vi "Nested Malleable VIs - Lesson 5.vi"() -> ()   [LabVIEW 2023]
doc: "Lesson 5 explores how creating nested VIMs can improve your code reuse, allowing many different malleable algorithms to be built around the same malleable core."
uses:
  Numeric Strings Less Functor/Numeric Strings Less Functor.lvclass
  e3db7b28-214a-4d56-9631-a08b30ab005c.vi
  c33f52e0-d72d-45e0-ba34-8b6af2d75d3b.vi
  2e45c285-a169-4a6c-a5e0-64cd902b0f72.vi
  f9130e0b-cd9d-4b76-83ef-857f5d1a4067.vi
  e3db7b28-214a-4d56-9631-a08b30ab005c.vi/4611cae3-c7be-41e2-9a5e-ea0ae78a7ced.vi
  c33f52e0-d72d-45e0-ba34-8b6af2d75d3b.vi/c0db33a9-eb6c-44d9-b982-8563e05d2734.vi
  c33f52e0-d72d-45e0-ba34-8b6af2d75d3b.vi/ae3535a8-0066-4e8d-a5de-b07ac05a7c65.vi
  c33f52e0-d72d-45e0-ba34-8b6af2d75d3b.vi/dda8e586-731b-4197-ad83-6a4d05585a0a.vi
  2e45c285-a169-4a6c-a5e0-64cd902b0f72.vi/4611cae3-c7be-41e2-9a5e-ea0ae78a7ced.vi
  f9130e0b-cd9d-4b76-83ef-857f5d1a4067.vi/d4db2432-cc9c-482c-8957-dac855435ef6.vi
  f9130e0b-cd9d-4b76-83ef-857f5d1a4067.vi/86fbf154-bd7b-49a2-8ab2-a837b2a95f24.vi
  f9130e0b-cd9d-4b76-83ef-857f5d1a4067.vi/3b95b01e-1ec2-4565-bcd9-7606a5281010.vi
  f9130e0b-cd9d-4b76-83ef-857f5d1a4067.vi/96a08935-737a-44b2-979c-a81d56408f7e.vi
  e3db7b28-214a-4d56-9631-a08b30ab005c.vi/4611cae3-c7be-41e2-9a5e-ea0ae78a7ced.vi/19e2e4cb-e3bb-4239-bd5f-680916605f5d.vi
  e3db7b28-214a-4d56-9631-a08b30ab005c.vi/4611cae3-c7be-41e2-9a5e-ea0ae78a7ced.vi/f72612c1-738a-48a1-9fcf-3db66cb27fb3.vi
  e3db7b28-214a-4d56-9631-a08b30ab005c.vi/4611cae3-c7be-41e2-9a5e-ea0ae78a7ced.vi/45406051-8994-464b-8b47-ac12a8cbadfa.vi
  e3db7b28-214a-4d56-9631-a08b30ab005c.vi/4611cae3-c7be-41e2-9a5e-ea0ae78a7ced.vi/dd886480-778c-48b1-8e4a-d6890e1a60dd.vi
  e3db7b28-214a-4d56-9631-a08b30ab005c.vi/4611cae3-c7be-41e2-9a5e-ea0ae78a7ced.vi/2e6e140f-e361-4312-a09e-e37273ac7fd1.vi
  e3db7b28-214a-4d56-9631-a08b30ab005c.vi/4611cae3-c7be-41e2-9a5e-ea0ae78a7ced.vi/3589548e-4c68-4568-af05-72ab28470577.vi
  e3db7b28-214a-4d56-9631-a08b30ab005c.vi/4611cae3-c7be-41e2-9a5e-ea0ae78a7ced.vi/cf64d4f5-91bd-4749-9577-68c6ded0155b.vi
  e3db7b28-214a-4d56-9631-a08b30ab005c.vi/4611cae3-c7be-41e2-9a5e-ea0ae78a7ced.vi/6f6fefe9-f25b-4595-b26f-75715299a794.vi
  e3db7b28-214a-4d56-9631-a08b30ab005c.vi/4611cae3-c7be-41e2-9a5e-ea0ae78a7ced.vi/c74ffb76-1048-4639-9a95-b6de96ba7014.vi
  2e45c285-a169-4a6c-a5e0-64cd902b0f72.vi/4611cae3-c7be-41e2-9a5e-ea0ae78a7ced.vi/19e2e4cb-e3bb-4239-bd5f-680916605f5d.vi
  2e45c285-a169-4a6c-a5e0-64cd902b0f72.vi/4611cae3-c7be-41e2-9a5e-ea0ae78a7ced.vi/f72612c1-738a-48a1-9fcf-3db66cb27fb3.vi
  2e45c285-a169-4a6c-a5e0-64cd902b0f72.vi/4611cae3-c7be-41e2-9a5e-ea0ae78a7ced.vi/45406051-8994-464b-8b47-ac12a8cbadfa.vi
  2e45c285-a169-4a6c-a5e0-64cd902b0f72.vi/4611cae3-c7be-41e2-9a5e-ea0ae78a7ced.vi/dd886480-778c-48b1-8e4a-d6890e1a60dd.vi
  2e45c285-a169-4a6c-a5e0-64cd902b0f72.vi/4611cae3-c7be-41e2-9a5e-ea0ae78a7ced.vi/2e6e140f-e361-4312-a09e-e37273ac7fd1.vi
  2e45c285-a169-4a6c-a5e0-64cd902b0f72.vi/4611cae3-c7be-41e2-9a5e-ea0ae78a7ced.vi/3589548e-4c68-4568-af05-72ab28470577.vi
  2e45c285-a169-4a6c-a5e0-64cd902b0f72.vi/4611cae3-c7be-41e2-9a5e-ea0ae78a7ced.vi/cf64d4f5-91bd-4749-9577-68c6ded0155b.vi
  2e45c285-a169-4a6c-a5e0-64cd902b0f72.vi/4611cae3-c7be-41e2-9a5e-ea0ae78a7ced.vi/6f6fefe9-f25b-4595-b26f-75715299a794.vi
  2e45c285-a169-4a6c-a5e0-64cd902b0f72.vi/4611cae3-c7be-41e2-9a5e-ea0ae78a7ced.vi/c74ffb76-1048-4639-9a95-b6de96ba7014.vi
  f9130e0b-cd9d-4b76-83ef-857f5d1a4067.vi/d4db2432-cc9c-482c-8957-dac855435ef6.vi/6eaecd13-6e48-4772-a921-b51ebdf84d88.vi
  f9130e0b-cd9d-4b76-83ef-857f5d1a4067.vi/d4db2432-cc9c-482c-8957-dac855435ef6.vi/d2d5f2b7-06f4-47f6-971c-049c3fdbb653.vi
  f9130e0b-cd9d-4b76-83ef-857f5d1a4067.vi/3b95b01e-1ec2-4565-bcd9-7606a5281010.vi/6eaecd13-6e48-4772-a921-b51ebdf84d88.vi
  f9130e0b-cd9d-4b76-83ef-857f5d1a4067.vi/3b95b01e-1ec2-4565-bcd9-7606a5281010.vi/d2d5f2b7-06f4-47f6-971c-049c3fdbb653.vi
  f9130e0b-cd9d-4b76-83ef-857f5d1a4067.vi/96a08935-737a-44b2-979c-a81d56408f7e.vi/6eaecd13-6e48-4772-a921-b51ebdf84d88.vi
  f9130e0b-cd9d-4b76-83ef-857f5d1a4067.vi/96a08935-737a-44b2-979c-a81d56408f7e.vi/d2d5f2b7-06f4-47f6-971c-049c3fdbb653.vi
  Numeric Strings Less Functor/Less Than.vi
panel:
  out "sorted array 3":string[](array[string])
  out "sorted array 2":string[](array[string])
  out "sorted array 1":string[](array[string])
  out "found":bool
  out "nearest index":i32
  # "Overview: This lesson explores how creating nested VIMs can improve your code reuse, allowing many different algorithms to be built around the same malleable core. \n\nInstructions: \n1. Open the block diagram of this VI. Review the lessons presented there.\n2. Run the VI to see the results. \n3. This lesson concludes this example."
  # "This array is sorted by string value, ignoring case."
  # "This array is sorted by string value, ignoring case."
  # "This array is sorted by the value of the number at the front, ignoring the rest of the string."
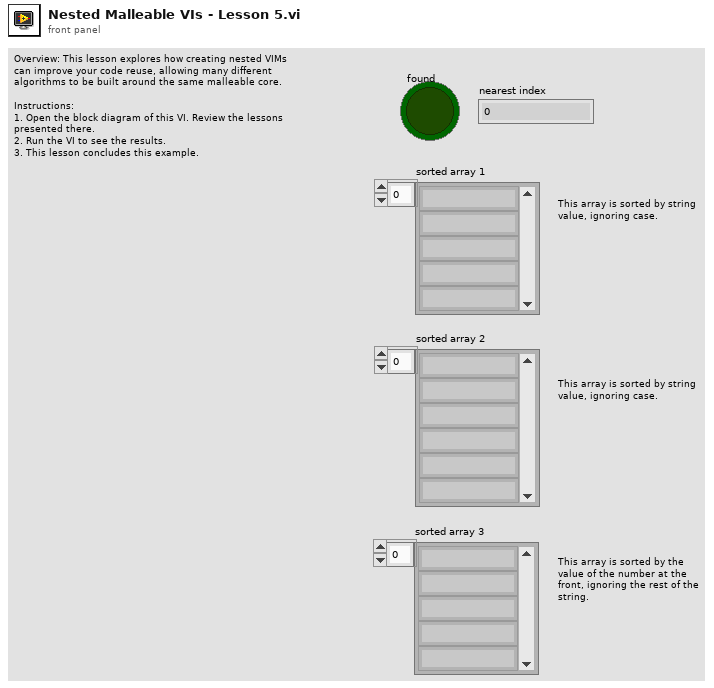
[diagram p1: front panel]
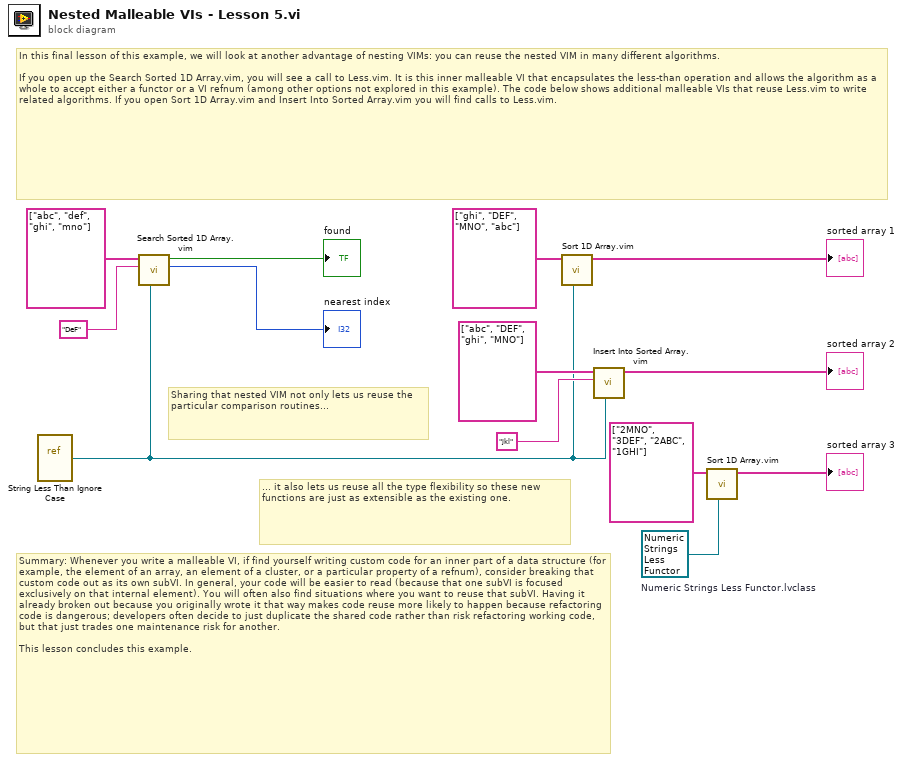
[diagram p0: block diagram]
diagram:
  w5 = refnum<class "Numeric Strings Less Functor.lvclass"> refnum  # Numeric Strings Less Functor.lvclass
  # "... it also lets us reuse all the type flexibility so these new functions are just as extensible as the existing one."
  # "Sharing that nested VIM not only lets us reuse the particular comparison routines..."
  # "Summary: Whenever you write a malleable VI, if find yourself writing custom code for an inner part of a data structure (for example, the element of an array, an element of a cluster, or a particular property of a refnum), consider breaking that custom code out as its own subVI. In general, your code will be easier to read (because that one subVI is focused exclusively on that internal element). You will often also find situations where you want to reuse that subVI. Having it already broken out because you originally wrote it that way makes code reuse more likely to happen because refactoring code is dangerous; developers often decide to just duplicate the shared code rather than risk refactoring working code, but that just trades one maintenance risk for another.\n\nThis lesson concludes this example."
  # "In this final lesson of this example, we will look at another advantage of nesting VIMs: you can reuse the nested VIM in many different algorithms.\n\nIf you open up the Search Sorted 1D Array.vim, you will see a call to Less.vim. It is this inner malleable VI that encapsulates the less-than operation and allows the algorithm as a whole to accept either a functor or a VI refnum (among other options not explored in this example). The code below shows additional malleable VIs that reuse Less.vim to write related algorithms. If you open Sort 1D Array.vim and Insert Into Sorted Array.vim you will find calls to Less.vim."
  n1 = vi-ref "String Less Than Ignore Case.vi"() -> (w1:refnum<vi>)
  n2 = call "Search Sorted 1D Array.vim"("less function (built-in <)"=w1, "element"="DeF", "sorted 1D array"=string[] ["abc", "def", "ghi", "mno"] ("1D array")) -> ("nearest index"=→"nearest index":i32, "found?"=→"found":bool)  [unwired: 7 in]
  n3 = call "Sort 1D Array.vim"("less function (built-in <)"=w1, "unsorted array"=string[] ["ghi", "DEF", "MNO", "abc"] ("1D array")) -> ("sorted array"=→"sorted array 1":string[])  [unwired: 9 in]
  n4 = call "Insert Into Sorted Array.vim"("less function (built-in <)"=w1, "element"="jkl", "sorted array in"=string[] ["abc", "DEF", "ghi", "MNO"] ("1D array")) -> ("sorted array out"=→"sorted array 2":string[])  [unwired: 8 in]
  n5 = call "Sort 1D Array.vim"("less function (built-in <)"=w5, "unsorted array"=string[] ["2MNO", "3DEF", "2ABC", "1GHI"] ("1D array")) -> ("sorted array"=→"sorted array 3":string[])  [unwired: 9 in]
